vi "handleRecord.vi"(8 "error in (no error)":errorcluster, 10 "Record":refnum<class "Record.lvclass">, 11 "Handler.File in":refnum<class "Handler.File.lvclass">) -> (0 "error out":errorcluster, 3 "Handler.File out":refnum<class "Handler.File.lvclass">)   [LabVIEW 2017, in "Error Log.lvlib" / "Handler.File.lvclass"]
uses:
  Handler.File.lvclass
  Record/Record.lvclass
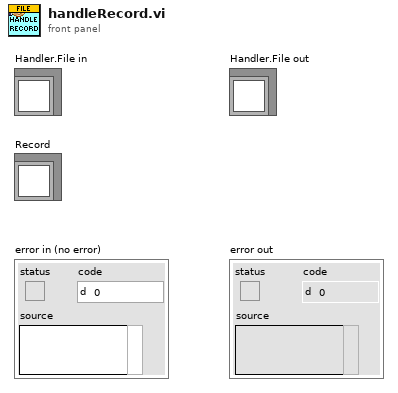
[diagram p1: front panel]
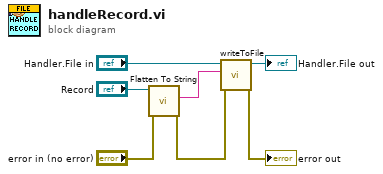
[diagram p0: block diagram]
diagram:
  n1 = call "Flatten To String.vi"("error in (no error)"="error in (no error)", "Record in"="Record") -> ("error out"=w2:errorcluster, "String"=w3:string)  [unwired: 7 in, 1 out]
  n2 = call-dynamic "writeToFile.vi"("error in (no error)"=w2, "New Record String"=w3, "Handler.File in"="Handler.File in") -> ("error out"=→"error out":errorcluster, "Handler.File out"=→"Handler.File out":refnum<class "Handler.File.lvclass">)  [unwired: 7 in]
